vi "Write Status.vi"(8 "error in (no error)":errorcluster, 10 "Status":T1, 11 "Socket in":refnum<class "Execution.lvclass">) -> (0 "error out":errorcluster, 3 "Socket out":refnum<class "Execution.lvclass">)   [LabVIEW 2015, in "Execution.lvclass"]
uses:
  Execution.lvclass
  EXECUTION_STATUS.ctl
  Execution.lvclass/Execution.ctl
  EXECUTION_UI_MSG.ctl
  Send UI Message.vi
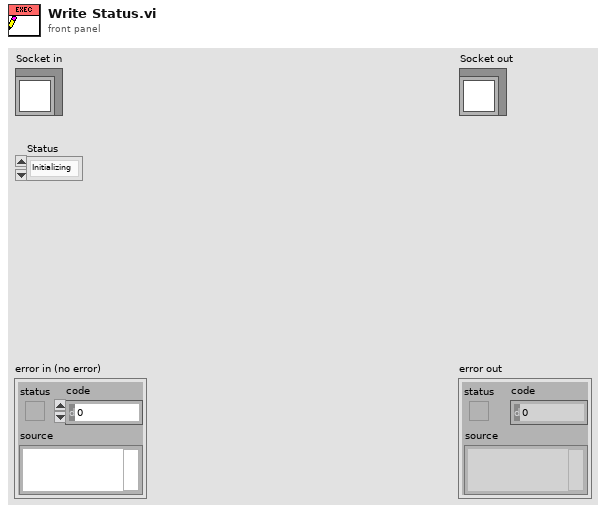
[diagram p1: front panel]
types:
  T1 = typedef "Execution.lvclass/EXECUTION_STATUS.ctl" = enum16{"Initializing ", "Disable", "Ready", "Running", "Finished"}
  T2 = typedef "Execution.lvclass/EXECUTION_UI_MSG.ctl" = enum16{"EXECUTION_STATUS", "INIT_UI", "DUT_UPDATE", "BOTTOM_PANEL_UPDATE", "TOP_PANEL_UPDATE", "STEP_START", "STEP_END", "DISPLAY_RESULT", "APPLICATION_END"}
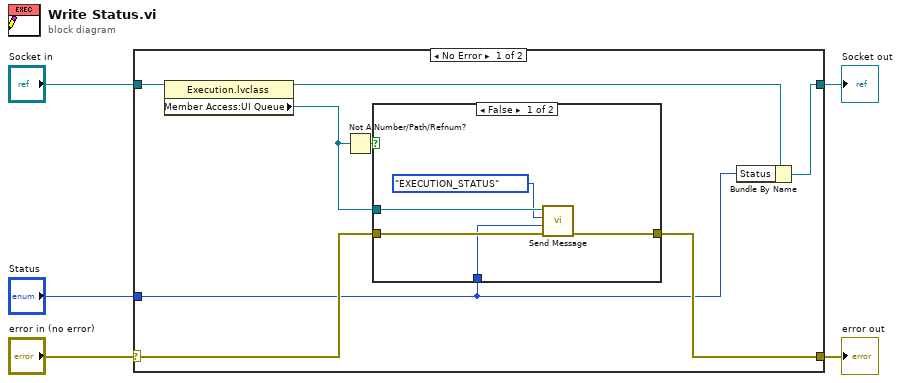
[diagram p0: block diagram]
diagram:
  n1 = case shown="No Error" "error in (no error)" {
    selector: "error in (no error)" -> [w8 w20]
    tunnel: [w7 w20] -> w4
    tunnel: [w13 w21] -> w2
    tunnel: "Socket in" -> [w12 w21]
    tunnel: "Status" -> [w6 _]
    frame No Error {
      n2 = property class="Execution.lvclass"(reference=w12) -> (reference out=w11:refnum<class "Execution.lvclass">, "Member Access:UI Queue"=w9:refnum<queue>)  [unwired: 1 in, 1 out]
      n3 = Not A Number/Path/Refnum?(number/path/refnum=w9) -> (NaN/Path/Refnum?=w10:bool)
      n4 = case shown="False" w10 {
        tunnel: w9 -> [w18 _]
        tunnel: w8 -> [w17 w19]
        tunnel: [w16 w19] -> w7
        tunnel: w6 -> [w15 _]
        frame False {
          n5 = call-poly "Send Message.vi"("error in (no error)"=w17, "Data"=w15, "Msg"=EXECUTION_UI_MSG."EXECUTION_STATUS", "UI Queue"=w18) -> ("error out"=w16:errorcluster)  [unwired: 7 in]
        }
        frame True {
        }
      }
      n6 = Bundle By Name(cluster=w11, "Status"=w6) -> (w13:refnum<class "Execution.lvclass">)
    }
    frame Error {
    }
  }
  "error out" <- w4
  "Socket out" <- w2
